vi "Get Class Name Enum.vi"(8 "error in (no error)":errorcluster, 11 "reference":refnum<vi>) -> (0 "error out":errorcluster, 3 "Enum":T1(ring))   [LabVIEW 2018, in "Scripting Tools.lvlib"]
uses:
  Scripting Tools.lvlib
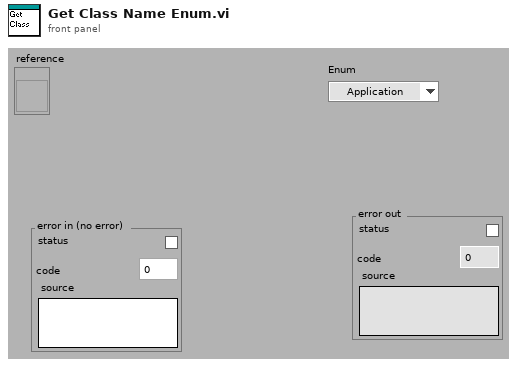
[diagram p1: front panel]
types:
  T1 = enum16{"Application", "VI", "PolymorphicVI", "MethodVI", "FacadeVI", "Generic", "FlatSequenceFrame", "TimeSequenceFrame", "SubWizard", "CodeWizard", "StateDiagramWizard", "MasterWizard", "Probe", "ConnectorPane", "Page", "Cursor", "Plot", "GObject", "TimedStructDCO", "SynchronousDataFlowDCO", "PolymorphicVISelector", "FlatSequenceOuterTunnel", "FlatSequenceInnerTunnel", "SimulationDCO", "FlatSequence", "TimeFlatSequence", "PropertyItem", "Wire", "SequenceLocal", "Tunnel", "SelectorTunnel", "LeftShiftRegister", "LoopTunnel", "RightShiftRegister", "Node", "TimedSequence", "XNode", "XDataNode", "StaticVIReference", "ControlReferenceConstant", "GrowableFunction", "Unbundler", "NamedUnbundler", "FormatScanString", "ObjectFunction", "Constructor", "Invoke", "Property", "CallLibrary", "CIN", "Bundler", "NamedBundler", "BuildArray", "IndexArray", "CompoundArithmetic", "BuildClusterArray", "Formula", "MathScriptNode", "ScriptNode", "Structure", "SynchronousDataFlowNode", "SimulationNode", "MultiFrameStructure", "DisableStructure", "EventStructure", "CaseStructure", "Sequence", "ExternalNode", "Loop", "WhileLoop", "TimedLoop", "ForLoop", "UnitCast", "CallByRef", "SubVI", "ConfNode", "PolymorphicSubVI", "Function", "FileDialog", "ArrayToCluster", "GPIBReadWrite", "FlattenUnflattenString", "FlattenString", "TypeCast", "ReadWriteFile", "Comparison", "Local", "Global", "FormulaParameter", "MathScriptNodeParameter", "ScriptNodeParameter", "Constant", "LabVIEWClassConstant", "AbsTimeConstant", "RefNumConstant", "ClassSpecifierConstant", "ColorBoxConstant", "IONameConstant", "GenClassTagFlatRefConstant", "GenClassTagRefConstant", "DAQmxNameConstant", "IVILogicalNameConstant", "VISAResourceNameConstant", "DAQChannelNameConstant", "DSCTagConstant", "BooleanConstant", "FixedConstant", "ClusterConstant", "StringConstant", "ComboBoxConstant", "NumericConstant", "NamedNumericConstant", "EnumConstant", "RingConstant", "DigitalNumericConstant", "ArrayConstant", "PathConstant", "Terminal", "OuterTerminal", "InnerTerminal", "ControlTerminal", "AbstractDiagram", "MathDiagram", "Diagram", "SDFCompanionDiagram", "SdfDiagram", "CompanionDiagram", "SimDiagram", "TopLevelDiagram", "Splitter", "Pane", "Scale", "SlideScale", "ColorGraphScale", "GraphScale", "ColorScale", "RotaryColorScale", "Panel", "Control", "LabVIEWClassControl", "SceneGraphDisplay", "Scrollbar", "Pixmap", "PlugInDDODummyContainer", "PlugInControl", "TreeControl", "SubPanel", "DigitalTable", "AbsTime", "PageSelector", "TabControl", "WaveformData", "MulticolumnListbox", "Cluster", "RadioButtonsControl", "IOName", "GenClassTagFlatRef", "GenClassTagRef", "DAQmxName", "IVILogicalName", "VISAResourceName", "DAQChannelName", "DSCTag", "String", "ComboBox", "GraphChart", "MixedSignalGraph", "IntensityGraph", "IntensityChart", "WaveformGraph", "DigitalGraph", "XYGraph", "WaveformChart", "Numeric", "NumericWithScale", "Knob", "Slide", "ColorRamp", "NamedNumeric", "Enum", "Ring", "Digital", "ActiveXContainer", "Picture", "Array", "Table", "ListBox", "Path", "LVVariant", "RefNum", "GenClassRef", "LVObjectRefNum", "VIRefNum", "TypedRefNum", "Boolean", "ColorBox", "Decoration", "Text", "NumericText", "Project", "ProjectItem", "PropertyFolder", "XPropertyFolder", "TargetItem", "Library", "XInterfaceLibrary", "XNodeLibrary", "XControlLibrary", "LVClassLibrary", "BuildSpecification", "Variable", "TagSet", "SceneWindow", "LVTarget", "Provider", "CopyOperation", "ProjectItemType", "CopyItem", "CopyConflict", "CopyExpert", "SceneNode", "SceneClipPlane", "SceneLight", "SceneObject", "SceneTexture", "SceneGeometry", "SceneMesh", "SceneSphere", "SceneHeightField", "SceneCylinder", "SceneCone", "SceneBox"}
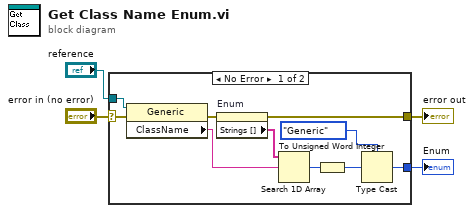
[diagram p0: block diagram]
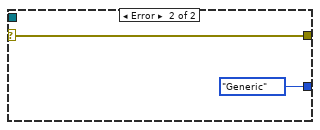
[diagram p2: hidden frame]
diagram:
  n1 = case shown="No Error" "error in (no error)" {
    selector: "error in (no error)" -> [w13 w16]
    tunnel: "reference" -> [w14 _]
    tunnel: [w6 T1."Generic" ("Enum")] -> w2
    tunnel: [w8 w16] -> w1
    frame No Error {
      n2 = property class="Generic"(reference=w14, error in=w13) -> (error out=w9:errorcluster, "ClassName"=w12:string)  [unwired: 1 out]
      n3 = property on="Enum" class="Enum (strict)"(error in=w9) -> (error out=w8:errorcluster, "Strings []"=w11:string[])  [unwired: 1 in, 1 out]
      n4 = Search 1D Array(1D array=w11, element=w12) -> (index of element=w10:i32)  [unwired: 1 out]
      n5 = To Unsigned Word Integer(number=w10) -> (unsigned 16bit integer=w7:u16)
      n6 = Type Cast(type=T1."Generic" ("Enum"), x=w7) -> (*(type *) &x=w6:T1)
    }
    frame Error {
    }
  }
  "Enum" <- w2
  "error out" <- w1
